vi "Controller Read Inputs.vi"(8 "error in (no error)":errorcluster, 9 "PS Status Variables":refnum<k21>[](array[refnum]), 10 "PS Reading Variables":refnum<k21>[](array[refnum]), 11 "BPM Variables":refnum<k21>[](array[refnum])) -> (0 "error out":errorcluster, 1 "PS Status (per PS Rack)":u8[](array[numeric]), 2 "PS Readings":dbl[](array[numeric]), 3 "BPM Readings":dbl[](array[numeric]))   [LabVIEW 2011, in "Controller VIs.lvlib"]
doc: "Read all input variables from the Acquisition and Actuation chassis."
uses:
  Controller VIs.lvlib
  Simulated Beam VIs/Simulated Beam Response.vi
  Simulated Beam VIs/Simulated PS Current.vi
  <vilib>/Analysis/baseanly.llb/A x Vector.vi
  Simulated Beam VIs.lvlib
  <vilib>/Analysis/NI_AALBase.lvlib
  <vilib>/ptbypt/NI_PtbyPt.lvlib
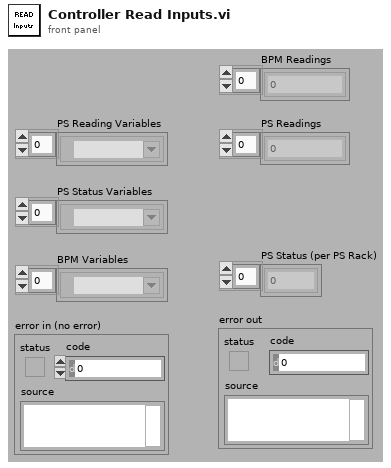
[diagram p1: front panel]
types:
  T1 = cluster{"filter structure":enum32{"IIR 2nd Order", "IIR 4th Order"}, "Reverse Coefficients":dbl[], "Forward Coefficients":dbl[]}
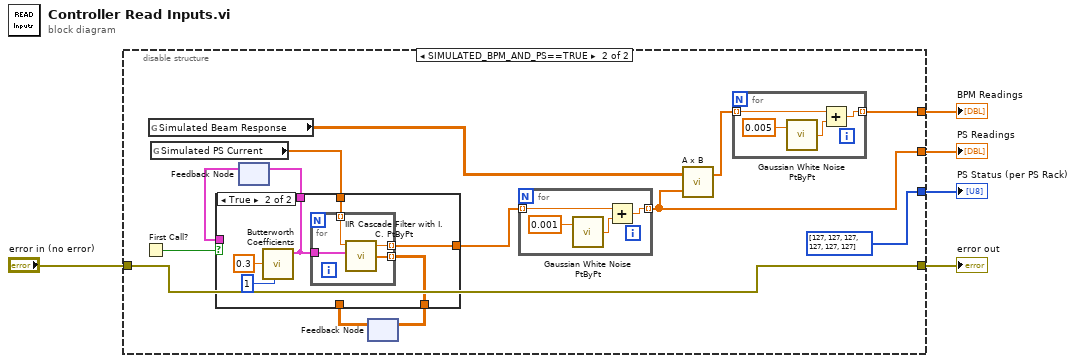
[diagram p0: block diagram]
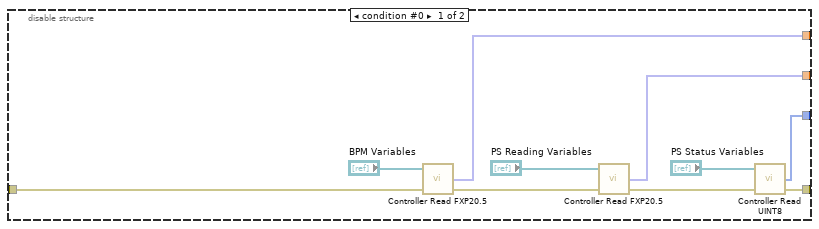
[diagram p2: hidden frame]
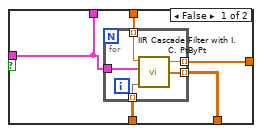
[diagram p3: hidden frame]
diagram:
  n1 = disable-structure shown="SIMULATED_BPM_AND_PS==TRUE" {
    disable-tunnel: [w15 w25] -> w5
    disable-tunnel: [w14 w23] -> w4
    disable-tunnel: [w13 u8[] [127, 127, 127, 127, 127, 127] ("PS Status (per PS Rack)")] -> w3
    disable-tunnel: "error in (no error)" -> [w9 w21]
    disable-tunnel: [w6 w21] -> w1
    frame condition #0 {
      n2 = call "Controller Read FXP20.5.vi"("error in (no error)"=w9, "Variables"="BPM Variables") -> ("error out"=w8:errorcluster, "Values"=w14:fxp<+/-,20,5>[])  [unwired: 2 in]
      n3 = call "Controller Read FXP20.5.vi"("error in (no error)"=w8, "Variables"="PS Reading Variables") -> ("error out"=w7:errorcluster, "Values"=w15:fxp<+/-,20,5>[])  [unwired: 2 in]
      n4 = call "Controller Read UINT8.vi"("error in (no error)"=w7, "Variables"="PS Status Variables") -> ("error out"=w6:errorcluster, "Values"=w13:u8[])  [unwired: 2 in]
    }
    frame condition #1 (active) {
      n5 = First Call?() -> (First Call?: T/F=w27:bool)
      n6 = global read "Simulated Beam Response.vi" "Simulated Beam Response"() -> (w28:dbl[][])
      n7 = global read "Simulated PS Current.vi" "Simulated PS Current"() -> (w20:dbl[])
      n8 = feedback #1() -> (w26:T1)  [unwired: 1 in]
      n9 = feedback #2() -> (w16:dbl[][])  [unwired: 1 in]
      n10 = case shown="True" w27 {
        tunnel: w26 -> [w34 _]
        tunnel: w20 -> [w33 w46]
        tunnel: [w34 w45] -> w19
        tunnel: [w37 w44] -> w18
        tunnel: [w36 w43] -> w17
        tunnel: w16 -> [w35 _]
        frame False {
          n11 = for {
            tunnel: w34 -> [w42]
            tunnel: [w41] -> w36 mode=indexing
            tunnel: [w40] -> w37 mode=indexing
            tunnel: w35 -> [w39] mode=indexing
            tunnel: w33 -> [w38] mode=indexing
            n12 = call <vilib>:"IIR Cascade Filter with I.C. PtByPt.vi"("x"=w38, "IIR Filter Cluster"=w42, "Initial Condition"=w39) -> ("Filtered x"=w40:dbl, "Final Condition"=w41:dbl[])  [unwired: 2 in, 1 out]
          }
        }
        frame True {
          n13 = call <vilib>:"Butterworth Coefficients.vi"("order"=1, "low cutoff freq: fl"=0.3) -> ("IIR Filter Cluster"=w45:T1)  [unwired: 8 in, 1 out]
          n14 = for {
            tunnel: w45 -> [w52]
            tunnel: [w51] -> w43 mode=indexing
            tunnel: w46 -> [w50] mode=indexing
            tunnel: [w49] -> w44 mode=indexing
            n15 = call <vilib>:"IIR Cascade Filter with I.C. PtByPt.vi"("x"=w50, "IIR Filter Cluster"=w52) -> ("Filtered x"=w49:dbl, "Final Condition"=w51:dbl[])  [unwired: 3 in, 1 out]
          }
        }
      }
      n16 = feedback-in #1(w19) -> ()
      n17 = feedback-in #2(w17) -> ()
      n18 = for {
        tunnel: [w55] -> w25 mode=indexing
        tunnel: w18 -> [w56] mode=indexing
        n19 = call <vilib>:"Gaussian White Noise PtByPt.vi"("standard deviation"=0.001 ("y")) -> ("Gaussian white noise"=w53:dbl)  [unwired: 2 in]
        n20 = Add(x=w56, y=w53) -> (x+y=w55:dbl)
      }
      n21 = call-poly <vilib>:"A x B.vi"("Vector"=w25, "A"=w28) -> ("A x Vector"=w22:dbl[])  [unwired: 1 out]
      n22 = for {
        tunnel: [w31] -> w23 mode=indexing
        tunnel: w22 -> [w32] mode=indexing
        n23 = call <vilib>:"Gaussian White Noise PtByPt.vi"("standard deviation"=0.005 ("y")) -> ("Gaussian white noise"=w29:dbl)  [unwired: 2 in]
        n24 = Add(x=w32, y=w29) -> (x+y=w31:dbl)
      }
    }
  }
  "BPM Readings" <- w4
  "PS Readings" <- w5
  "PS Status (per PS Rack)" <- w3
  "error out" <- w1
